vi "LinearSystemLoop_FlyWheel_Execute.vi"(5 "FlyWheelSim_Model _Params":T2={"DCMOTOR_TYPES"=enum."NEO", "Num Motors"=1, "Gearing"=128.0, "MOI kgm2"=26.0} {"MOI kgm2" format="%#_13g"; "Gearing" format="%#_13g"}, 7 "LinearSystem_FlyWheel_Ctrl_Params":T1={"Vel Model Std Dev Rad/Sec"=0.8, "Vel Meas Std Dev Rad/Sec"=0.02, "Vel Ctrl Tol Rad/Sec"=0.8, "Max Ctrl Out V"=12.0}, 8 "dT Sec":dbl=0.02, 10 "Velocity (Rad/Sec)\n(PV)":dbl, 11 "Velocity (Rad/Sec)\nSetpoint (SP)":dbl) -> (0 "Error":bool, 2 "Kalman FIltered\nVelocity (PV)":dbl, 3 "Motor Dmd":dbl)   [LabVIEW 2019, in "Trajectory_Library.lvlib"]
uses:
  TypeDef/LINEAR_SYSTEM_LOOP.ctl
  TypeDef/LINEAR_QUADRATIC_REGULATOR.ctl
  <vilib>/Analysis/Matrix/Datatypes/RealMatrix.ctl
  TypeDef/LINEAR_PLANT_INV_FF.ctl
  TypeDef/KALMAN_FILTER.ctl
  TypeDef/LINEAR_SYSTEM.ctl
  TypeDef/LINEAR_SYSTEM_ID_FLYWHEEL_MODEL.ctl
  Enum/DCMOTOR_TYPES_ENUM.ctl
  TypeDef/LINEAR_SYSTEM_LOOP_FLYWHEEL_CTRL_PARAMS.CTL
  MatBuilder_Create.vi
  DCMotor_GetCIM.vi
  DCMotor_GetAndymark9015.vi
  DCMotor_GetAndymarkRs775_125.vi
  DCMotor_GetBag.vi
  DCMotor_GetBanebotsRs550.vi
  DCMotor_GetBanebotsRs775.vi
  DCMotor_GetFalcon500.vi
  DCMotor_GetMiniCIM.vi
  DCMotor_GetNEO.vi
  DCMotor_GetNEO550.vi
  DCMotor_GetRomiBuiltIn.vi
  DCMotor_GetVex775Pro.vi
  DCMotor_GetAndymarkAM2235A.vi
  DCMotor_GetAndymarkAM3493.vi
  LinearSystem_New.vi
  MatrixHelper_Zero.vi
  MatBuilder_Fill.vi
  Matrix_Ident.vi
  DCMotor_New.vi
  Units_RotationsPerMinuteToRadiansPerSecond.vi
  MatrixHelper_CoerceSize.vi
  <vilib>/Analysis/7linalg.llb/Create Special Matrix.vi
  <vilib>/Analysis/7linalg.llb/Create Special Real Matrix.vi
  Trajectory_Library.lvlib
  <vilib>/Analysis/Matrix/NI_Matrix.lvlib
panel:
  out "out Linear System Loop":T4
  # "<States,1>"
  # "<FUTURE --- CLAMP TYPE -- For now\nuse Normalize>"
  # "Steady State Gain  \n<States,Outputs>"
  # "State Estimate <Statess,1>"
  # "<States,States>"
  # "<States,Inputs>"
  # "<Outputs,States>"
  # "<Outputs,Inputs>"
  # "<States,1>"
  # "<Inputs,1>"
  # "<States,Inputs>"
  # "<States,States>"
  # "Ref State <States,1>"
  # "Comp and capped \noutput <Inputs,1>"
  # "Controller gain\n<Inputs,States>"
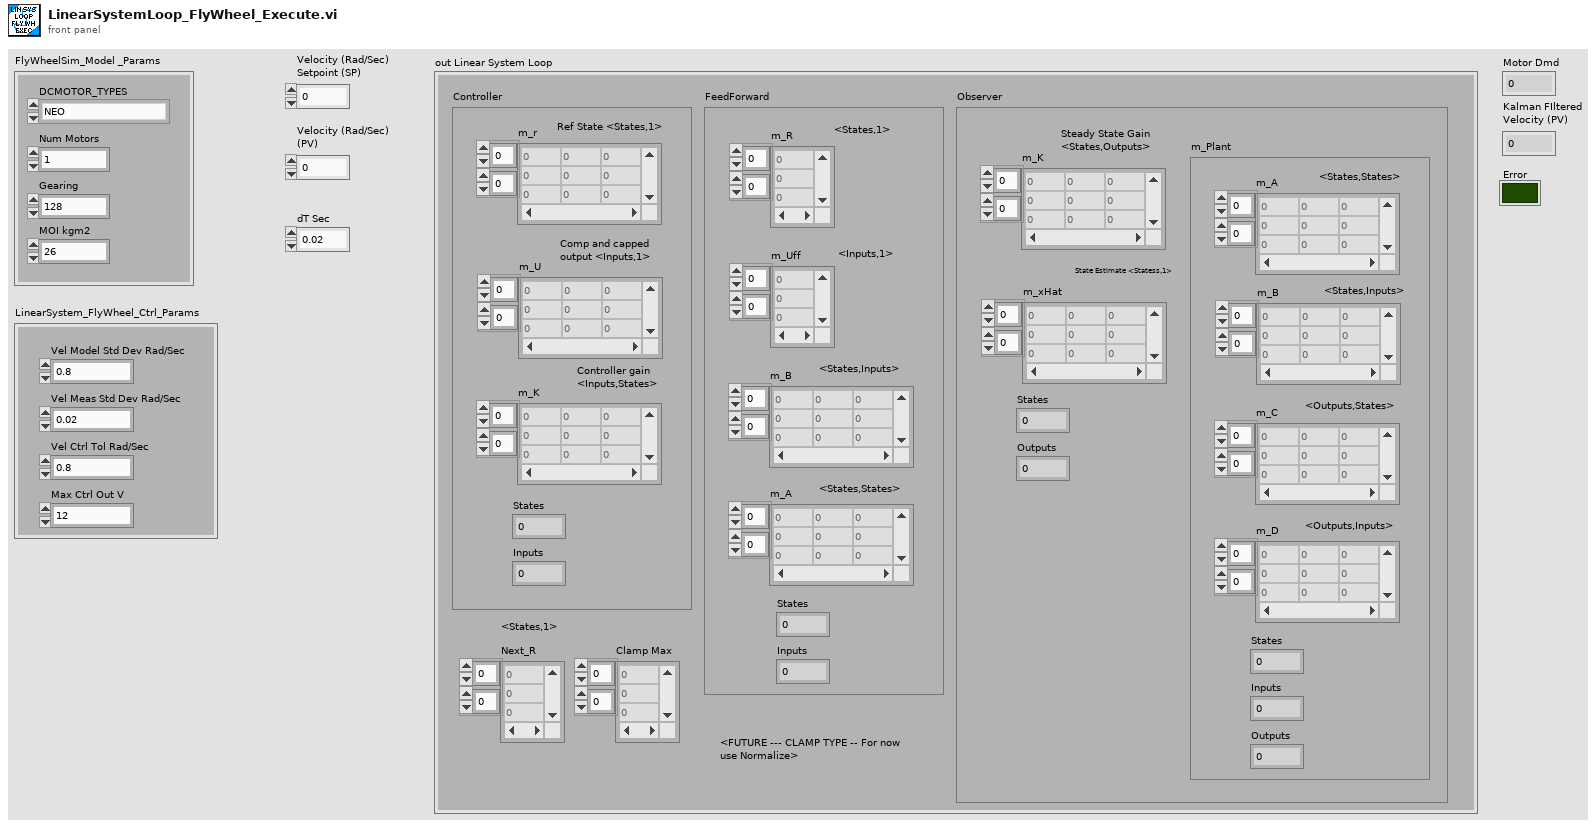
[diagram p1: front panel]
types:
  T1 = typedef "Trajectory_Library.lvlib/LINEAR_SYSTEM_LOOP_FLYWHEEL_CTRL_PARAMS.CTL" = cluster{"Vel Model Std Dev Rad/Sec":dbl, "Vel Meas Std Dev Rad/Sec":dbl, "Vel Ctrl Tol Rad/Sec":dbl, "Max Ctrl Out V":dbl}
  T2 = typedef "Trajectory_Library.lvlib/LINEAR_SYSTEM_ID_FLYWHEEL_MODEL.ctl" = cluster{"DCMOTOR_TYPES":T3, "Num Motors":i32, "Gearing":dbl, "MOI kgm2":dbl}
  T3 = typedef "Trajectory_Library.lvlib/DCMOTOR_TYPES_ENUM.ctl" = enum16{"CIM", "AndyMark 9015", "Andy Mark RS 775 125", "Bag", "BaneBots RS 550", "BaneBots RS 775", "Falcon 500", "Mini CIM", "NEO", "NEO 550", "Romi BuiltIn", "Vex 775 Pro", "Snow Blower AM 2235A", "Bosch Seat AM 3493"}
  T4 = typedef "Trajectory_Library.lvlib/LINEAR_SYSTEM_LOOP.ctl" = cluster{"Controller":T5, "FeedForward":T7, "Observer":T8, "Next_R":T6, "Clamp Max":T6}
  T5 = typedef "Trajectory_Library.lvlib/LINEAR_QUADRATIC_REGULATOR.ctl" = cluster{"m_r":T6, "m_U":T6, "m_K":T6, "States":i32, "Inputs":i32}
  T6 = typedef "NI_Matrix.lvlib/RealMatrix.ctl" = dbl[][]
  T7 = typedef "Trajectory_Library.lvlib/LINEAR_PLANT_INV_FF.ctl" = cluster{"m_R":T6, "m_Uff":T6, "m_B":T6, "m_A":T6, "States":i32, "Inputs":i32}
  T8 = typedef "Trajectory_Library.lvlib/KALMAN_FILTER.ctl" = cluster{"m_K":T6, "m_xHat":T6, "States":i32, "Outputs":i32, "m_Plant":T9}
  T9 = typedef "Trajectory_Library.lvlib/LINEAR_SYSTEM.ctl" = cluster{"m_A":T6, "m_B":T6, "m_C":T6, "m_D":T6, "States":i32, "Inputs":i32, "Outputs":i32}
  T10 = typedef "Trajectory_Library.lvlib/DCMOTOR.CTL" = cluster{"nominalVoltage_Volts":dbl, "StallTorque_NM":dbl, "StallCurrent_Amps":dbl, "FreeCurrent_Amps":dbl, "FreeSpeed_RadPerSec":dbl, "R_Ohms":dbl, "KvINV_RadPerSecPerVolt":dbl, "Kt_NMPerAmp":dbl, "L_H":dbl, "Jr_KgM2":dbl}
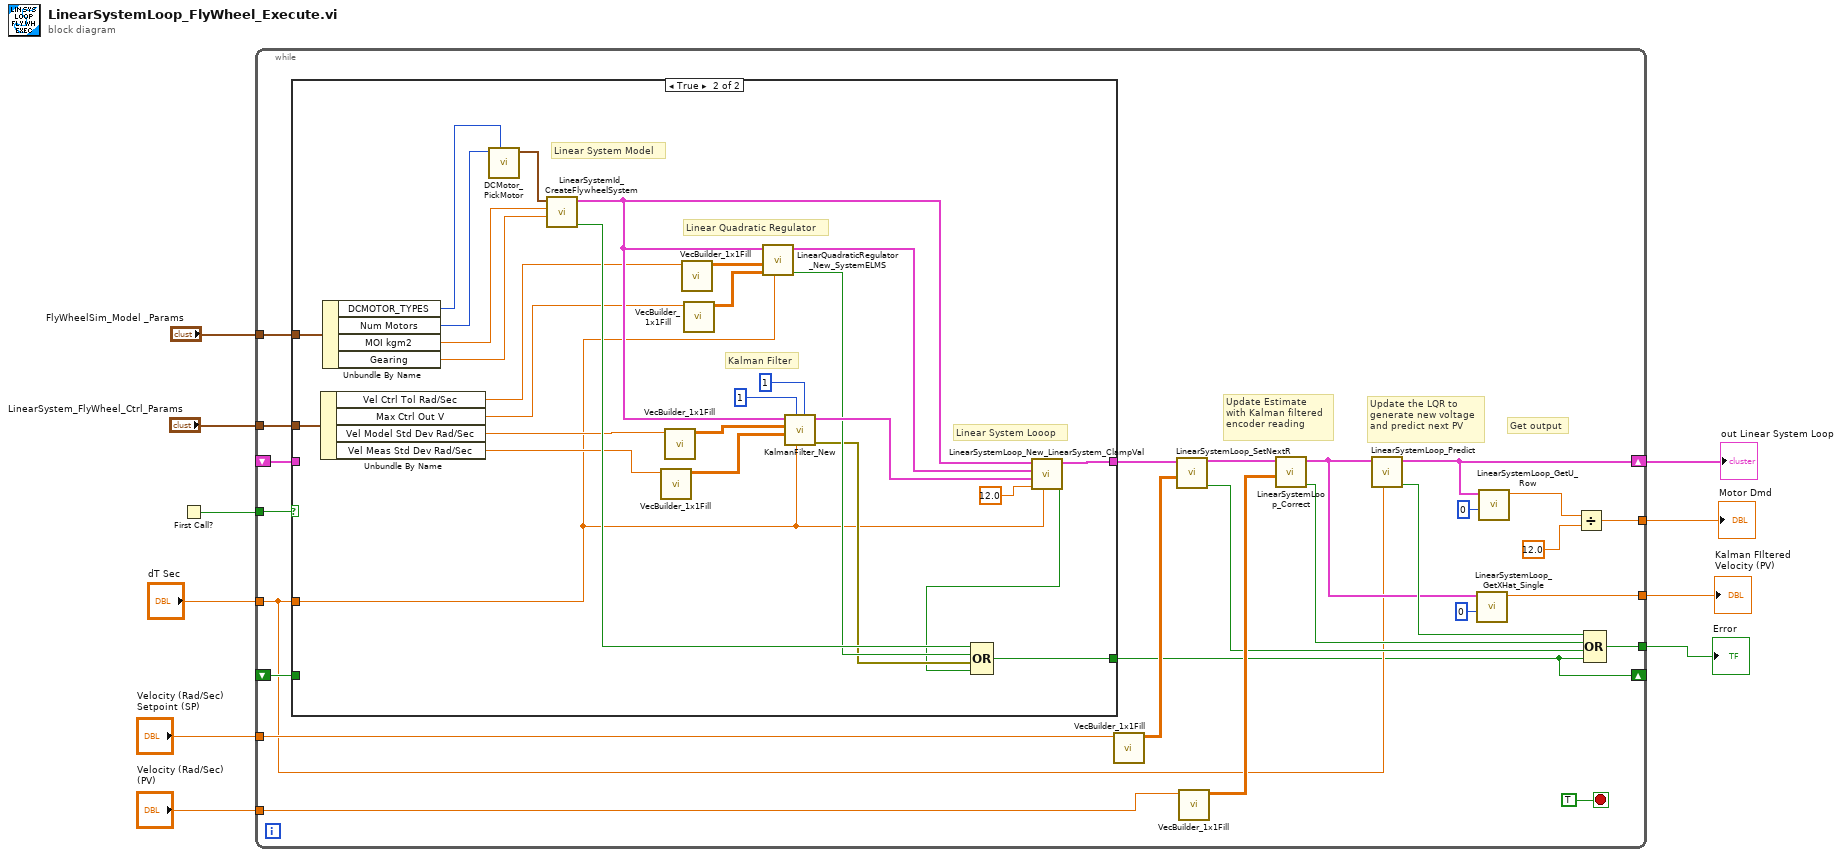
[diagram p0: block diagram]
diagram:
  n1 = First Call?() -> (First Call?: T/F=w5:bool)
  n2 = while {
    tunnel: "Velocity (Rad/Sec)\n(PV)" -> [w36]
    tunnel: [w19] -> w9
    tunnel: [w30] -> w8
    tunnel: "Velocity (Rad/Sec)\nSetpoint (SP)" -> [w26]
    shift-right: [w29] -> w7
    shift-left: _ -> [w23]
    tunnel: w5 -> [w18]
    tunnel: "FlyWheelSim_Model _Params" -> [w17]
    tunnel: "LinearSystem_FlyWheel_Ctrl_Params" -> [w15]
    shift-right: [w11] -> _
    shift-left: _ -> [w14]
    tunnel: "dT Sec" -> [w13]
    tunnel: [w12] -> w1
    stop <- TRUE stop-if-true
    # "Get output"
    # "Update the LQR to \ngenerate new voltage\nand predict next PV"
    # "Update Estimate\nwith Kalman filtered\nencoder reading"
    n3 = case shown="True" w18 {
      tunnel: w23 -> [w38 _]
      tunnel: [w38 w55] -> w22
      tunnel: w17 -> [_ w54]
      tunnel: [w37 w45] -> w11
      tunnel: w15 -> [_ w44]
      tunnel: w14 -> [w37 _]
      tunnel: w13 -> [_ w39]
      frame False {
      }
      frame True {
        # "Linear System Model"
        # "Linear System Looop"
        # "Linear Quadratic Regulator"
        # "Kalman Filter"
        n4 = Unbundle By Name(w44) -> ("Vel Ctrl Tol Rad/Sec"=w43:dbl, "Max Ctrl Out V"=w42:dbl, "Vel Model Std Dev Rad/Sec"=w41:dbl, "Vel Meas Std Dev Rad/Sec"=w40:dbl)
        n5 = Unbundle By Name(w54) -> ("DCMOTOR_TYPES"=w53:T3, "Num Motors"=w52:i32, "MOI kgm2"=w51:dbl, "Gearing"=w50:dbl)
        n6 = call "DCMotor_PickMotor.vi"("DCMOTOR_TYPES"=w53, "Num Motors"=w52) -> ("DCMOTOR"=w57:T10)  [unwired: 9 in]
        n7 = call "LinearSystemId_CreateFlywheelSystem.vi"("G"=w50, "jKgMetersSquared"=w51, "DCMOTOR"=w57) -> ("Error"=w49:bool, "Linearsystem"=w56:T9)  [unwired: 7 in]
        n8 = call "VecBuilder_1x1Fill.vi"("R0_C0"=w40) -> ("output matrix"=w63:T6)  [unwired: 10 in]
        n9 = call "VecBuilder_1x1Fill.vi"("R0_C0"=w41) -> ("output matrix"=w62:T6)  [unwired: 10 in]
        n10 = call "VecBuilder_1x1Fill.vi"("R0_C0"=w43) -> ("output matrix"=w58:T6)  [unwired: 10 in]
        n11 = call "VecBuilder_1x1Fill.vi"("R0_C0"=w42) -> ("output matrix"=w59:T6)  [unwired: 10 in]
        n12 = call "LinearQuadraticRegulator_New_SystemELMS.vi"("dt_Seconds"=w39, "Relms"=w59, "Qelms"=w58, "LINEARSYSTEM"=w56) -> ("Error"=w48:bool, "LinearQuadraticRegulator"=w64:T5)  [unwired: 6 in]
        n13 = call "KalmanFilter_New.vi"("States"=1, "dt_Seconds"=w39, "Outputs"=1, "MeasurementStdDevs"=w63, "StateStdDevs"=w62, "Plant"=w56) -> ("Error"=w47:errorcluster, "KalmanFilter"=w65:T8)  [unwired: 4 in]
        n14 = call "LinearSystemLoop_New_LinearSystem_ClampVal.vi"("dT_Seconds"=w39, "Max_Voltage"=12.0, "Observer"=w65, "Controller"=w64, "Plant"=w56) -> ("Error"=w46:bool, "Linear System Loop"=w55:T4)  [unwired: 5 in]
        n15 = Compound Arithmetic op=OR(w49, w48, w47, w46) -> (w45:bool)
      }
    }
    n16 = call "VecBuilder_1x1Fill.vi"("R0_C0"=w26) -> ("output matrix"=w25:T6)  [unwired: 10 in]
    n17 = call "LinearSystemLoop_SetNextR.vi"("R"=w25, "input inear System Loop"=w22) -> ("Size Coerced"=w16:bool, "out Linear System Loop"=w33:T4)  [unwired: 8 in]
    n18 = call "VecBuilder_1x1Fill.vi"("R0_C0"=w36) -> ("output matrix"=w34:T6)  [unwired: 10 in]
    n19 = call "LinearSystemLoop_Correct.vi"("Y"=w34, "input inear System Loop"=w33) -> ("Error"=w27:bool, "out Linear System Loop"=w21:T4)  [unwired: 8 in]
    n20 = call "LinearSystemLoop_Predict.vi"("dT_Seconds"=w13, "input inear System Loop"=w21) -> ("Error"=w28:bool, "out Linear System Loop"=w29:T4)  [unwired: 8 in]
    n21 = call "LinearSystemLoop_GetXHat_Single.vi"("Row"=0, "input inear System Loop"=w21) -> ("XHat"=w19:dbl)  [unwired: 9 in]
    n22 = call "LinearSystemLoop_GetU_Row.vi"("Row"=0, "input inear System Loop"=w29) -> ("U"=w31:dbl)  [unwired: 9 in]
    n23 = Divide(x=w31, y=12.0) -> (x/y=w30:dbl)
    n24 = Compound Arithmetic op=OR(w28, w27, w16, w11) -> (w12:bool)
  }
  "Motor Dmd" <- w8
  "out Linear System Loop" <- w7
  "Error" <- w1
  "Kalman FIltered\nVelocity (PV)" <- w9
